vi "Initial Settings User Prompt.vi"(8 "error in (no error)":errorcluster) -> (0 "error out":errorcluster, 2 "Path out":path, 3 "Initial Settings":T1)   [LabVIEW 2019, in "Instrument Addon System Explorer.lvlib"]
uses:
  Instrument Addon System Explorer.lvlib
  Types/Initial User Selection.ctl
  Shared/Instrument Addon Shared.lvlib
panel:
  in  "OK":bool
  in  "Path":path caption="Previous Personality Path (Optional)"
  in  "Protocol":string(combo)
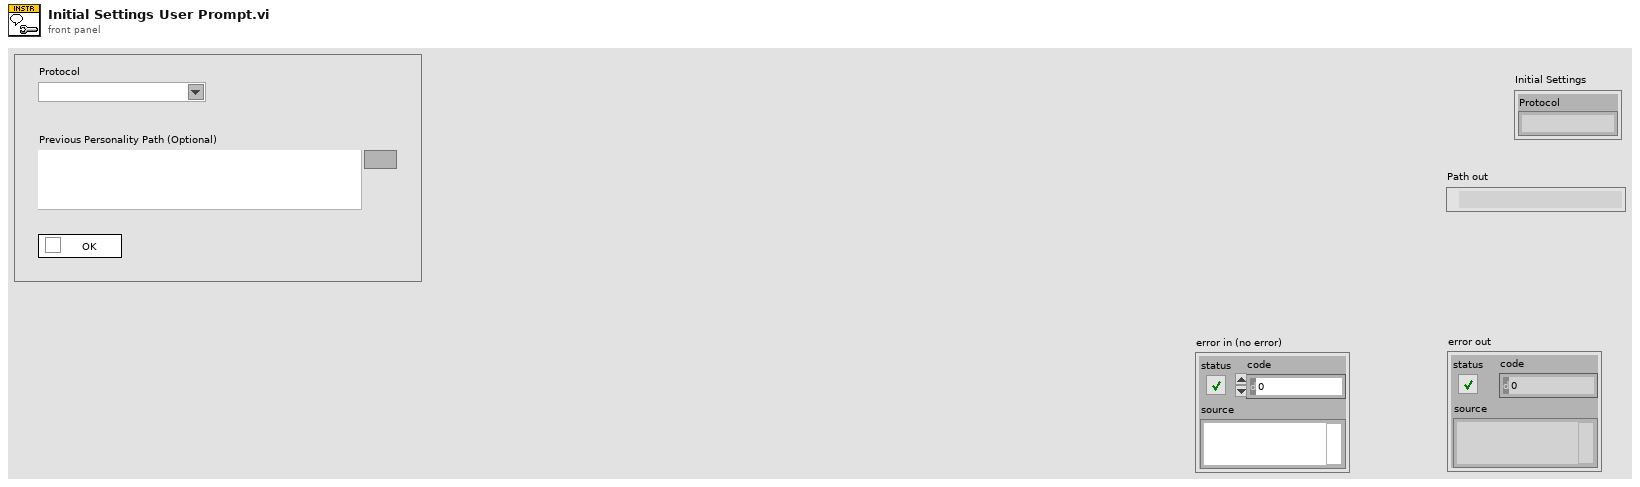
[diagram p1: front panel]
types:
  T1 = typedef "Instrument Addon System Explorer.lvlib/Initial User Selection.ctl" = cluster{"Protocol":string}
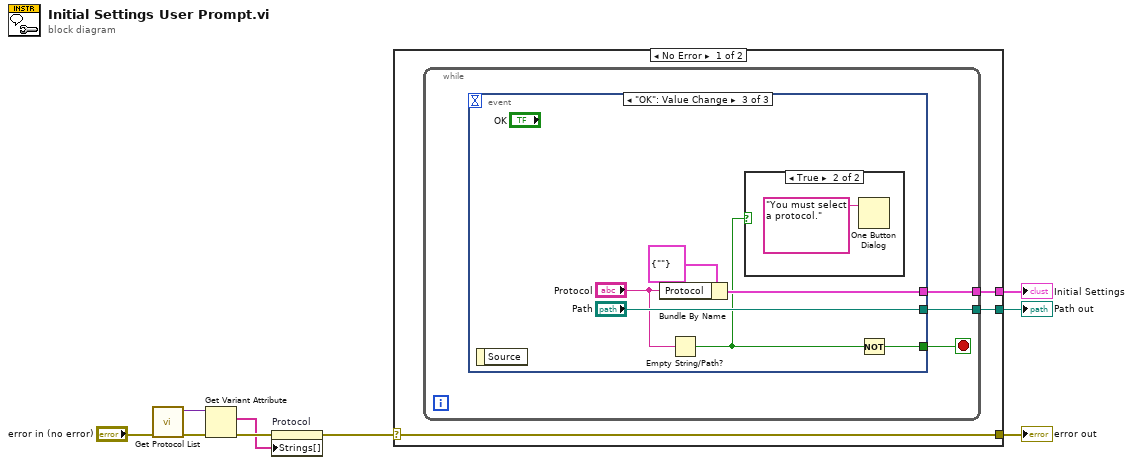
[diagram p0: block diagram]
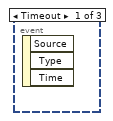
[diagram p2: hidden frame]
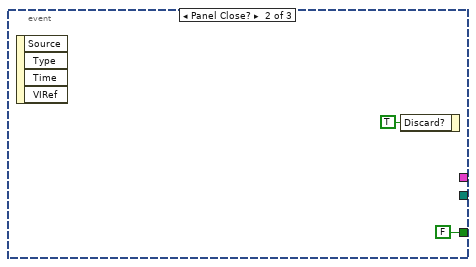
[diagram p3: hidden frame]
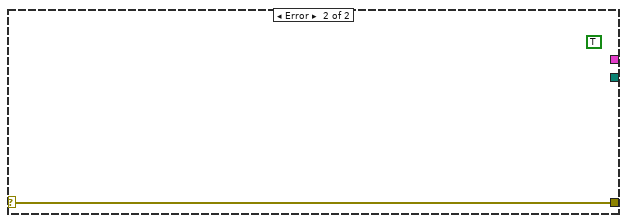
[diagram p5: hidden frame]
diagram:
  n1 = call "Get Protocol List.vi"("error in (no error)"="error in (no error)") -> ("error out"=w4:errorcluster, "Class Lookup"=w5:variant)  [unwired: 9 in]
  n2 = Get Variant Attribute(Variant=w5, error in=w4) -> (names=w1:string[], error out=w3:errorcluster)  [unwired: 2 in, 2 out]
  n3 = property on="Protocol" class="CmbBox"(error in=w3, "Strings[]"=w1) -> (error out=w2:errorcluster)  [unwired: 1 in, 1 out]
  n4 = case shown="No Error" w2 {
    selector: w2 -> [w10 w25]
    tunnel: [w12 _] -> w9
    tunnel: [w11 _] -> w8
    tunnel: [w10 w25] -> w7
    frame No Error {
      n5 = while {
        tunnel: [w15] -> w12
        tunnel: [w14] -> w11
        stop <- w13 stop-if-true
        n6 = event shown="[2] \"OK\": Value Change" {
          selector: _ -> [_ _ _]
          dyn-events: _ -> [_ _ _]
          timeout: _ -> [_ _ _]
          tunnel: [_ _ w22] -> w15
          tunnel: [_ _ "Path"] -> w14
          tunnel: [_ FALSE ("Discard?") w19] -> w13
          event Timeout {
            n7 = event-data() -> ()  [unwired: 1 in, 3 out]
          }
          event Panel Close? {
            n8 = event-data() -> ()  [unwired: 1 in, 4 out]
            n9 = event-data("Discard?"=TRUE) -> ()  [unwired: 1 in, 1 out]
          }
          event "OK": Value Change {
            n10 = event-data() -> ()  [unwired: 1 in, 1 out]
            n11 = Bundle By Name(cluster=T1 {"Protocol"=""}, "Protocol"="Protocol") -> (w22:T1)
            n12 = Empty String/Path?(string/path="Protocol") -> (empty?=w18:bool)
            n13 = case shown="True" w18 {
              frame False {
              }
              frame True {
                n14 = One Button Dialog(message="You must select a protocol.") -> ()  [unwired: 1 in, 1 out]
              }
            }
            n15 = Not(x=w18) -> (.not. x?=w19:bool)
          }
        }
      }
    }
    frame Error {
      (unwired) TRUE ("Discard?")
    }
  }
  "Initial Settings" <- w9
  "error out" <- w7
  "Path out" <- w8
